vi "Set Notifier Ref.vi"(8 "error in (no error)":errorcluster, 10 "notifier in":refnum<notifier>, 11 "CVT_I32 in":refnum<class "CVT_I32.lvclass">) -> (0 "error out":errorcluster, 3 "CVT_I32 out":refnum<class "CVT_I32.lvclass">)   [LabVIEW 2024, in "Current Value Table.lvlib" / "CVT_I32.lvclass"]
uses:
  CVT_I32.lvclass
  CVT_I32.lvclass/CVT_I32.ctl
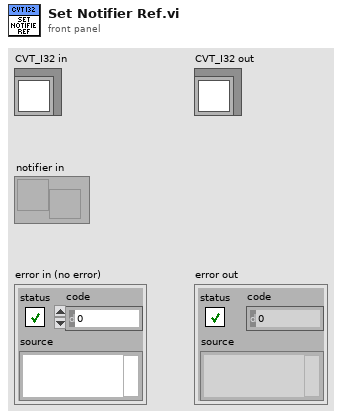
[diagram p1: front panel]
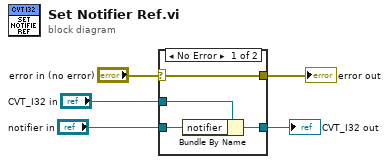
[diagram p0: block diagram]
diagram:
  n1 = case shown="No Error" "error in (no error)" {
    selector: "error in (no error)" -> [w8 w11]
    tunnel: [w8 w11] -> w4
    tunnel: [w7 w10] -> w2
    tunnel: "CVT_I32 in" -> [w9 w10]
    tunnel: "notifier in" -> [w6 _]
    frame No Error {
      n2 = Bundle By Name(cluster=w9, "notifier"=w6) -> (w7:refnum<class "CVT_I32.lvclass">)
    }
    frame Error {
    }
  }
  "error out" <- w4
  "CVT_I32 out" <- w2
